vi "Add Sink.vi"(8 "error in (no error)":errorcluster, 10 "Sink Name":string, 11 "Log Sink Reference":refnum<data-value>) -> (0 "error out":errorcluster)   [LabVIEW 2016, in "Stream Log.lvlib" / "Global Application Log.lvclass"]
doc: "--\nCopyright © 2017 Composed SystemsI All rights reserved.\n\nAuthor: Jon McBee <jon.mcbee@composed.io>\n\nThis library is provided \"AS IS\" ,WITHOUT WARRANTIES OR\nCONDITIONS OF ANY KIND, either express or implied.\n\nComposed Systems -- composed.io\n\nStream 0.0.1.1\nJon McBee - Composed Systems\nCopyright (c) 2017, Composed Systems"
uses:
  <userlib>/Composed Systems/Stream/Log/Global Application Log/Global Application Log.lvclass
  <userlib>/Composed Systems/Stream/Log/Log Sink/Log Sink.lvclass
  <userlib>/Composed Systems/Stream/Log/Global Application Log/Global Application Log.lvclass/Global Application Log.ctl
  <userlib>/Composed Systems/Stream/Log/Application Log/Application Log.lvclass
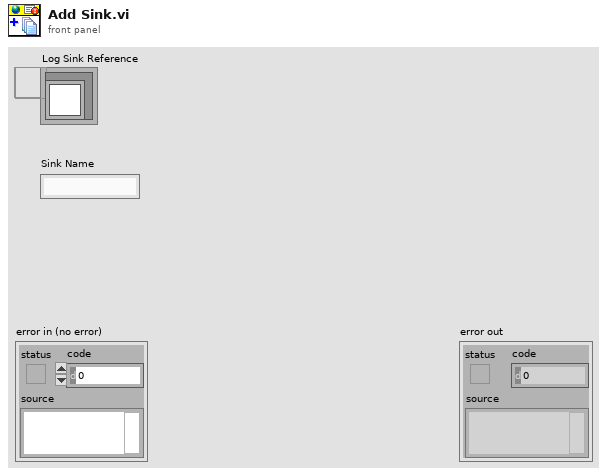
[diagram p1: front panel]
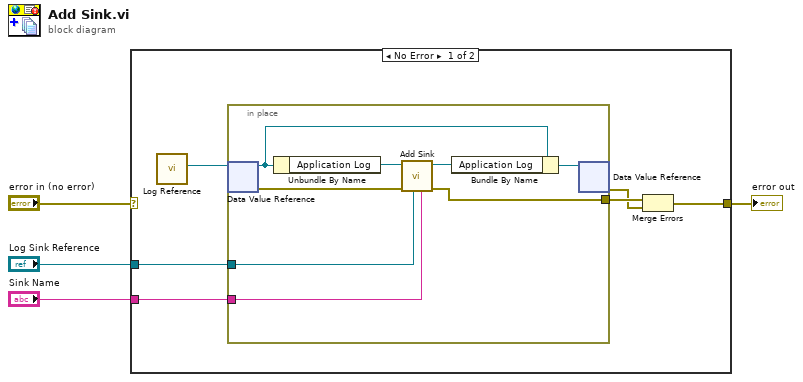
[diagram p0: block diagram]
diagram:
  n1 = case shown="No Error" "error in (no error)" {
    selector: "error in (no error)" -> [_ w19]
    tunnel: [w7 w19] -> w3
    tunnel: "Log Sink Reference" -> [w6 _]
    tunnel: "Sink Name" -> [w5 _]
    frame No Error {
      n2 = call <userlib>:"Log Reference.vi"() -> ("Global Log Reference out"=w10:refnum<data-value>)  [unwired: 11 in]
      n3 = in-place {
        in-place-border: [w13] -> w9
        in-place-border: w6 -> [w12]
        in-place-border: w5 -> [w11]
        n4 = in-place-dvr #1(w10) -> (w18:refnum<class "Global Application Log.lvclass">, w14:errorcluster)
        n5 = Unbundle By Name(w18) -> ("Application Log"=w16:refnum<class "Application Log.lvclass">)
        n6 = call <userlib>:"Add Sink.vi"("Sink Name"=w11, "Log Sink Reference"=w12, "error in (no error)"=w14, "Application Log in"=w16) -> ("error out"=w13:errorcluster, "Application Log out"=w15:refnum<class "Application Log.lvclass">)  [unwired: 6 in]
        n7 = Bundle By Name(cluster=w18, "Application Log"=w15) -> (w17:refnum<class "Global Application Log.lvclass">)
        n8 = in-place-dvr #1(w17) -> (w8:errorcluster)  [unwired: 1 out]
      }
      n9 = Merge Errors(w9, w8) -> (w7:errorcluster)
    }
    frame Error {
    }
  }
  "error out" <- w3
